vi "ZE_Recorder_InitializeTask.vi"(8 "error in (no error)":errorcluster, 9 "Sampling Rate [Hz]":dbl, 10 "Multi devices?":bool=TRUE, 11 "Channel Array in":T1 caption="Channel Array" {"Terminal" items=["Default"=-1, "RSE"=10083, "NRSE"=10078, "Differential"=10106, "Pseudodifferential"=12529]}) -> (0 "error out":errorcluster, 2 "Array":refnum<k21>[](array[refnum]), 3 "max Range":dbl)   [LabVIEW 2025, in "ZE_Recorder.lvlib"]
doc: "ZE_Recorder_InitializeTask.vi\n----------------------------------------------\nThis VI initalizes the necessary numbers of tasks accrding the number of devices used and assigns a common colck. It returns an array of tasks.\n\nInputs:\n---------------------\n- error in (no error) : Cluster; \n- Sampling Rate [Hz] : DBL; \n- Multi devices? : Boolean; \n- Channel Array : 1DArrayOfCluster; \n\nOutputs:\n---------------------\n- error out : Cluster; \n- Array : 1DArrayOfRefnum; \n- max Range : DBL; \n\n----------------------------------------------\n25.12.2016\nZühlke Engineering AG\nCH-8952 Schlieren\nwww.zuehlke.com"
uses:
  ZE_Recorder.lvlib
  ZE_Recorder_ChannelCluster.ctl
  ChannelCluster.ctl
  ZE_Recorder_Units.ctl
  Temperature.ctl
  <vilib>/DAQmx/configure/timing.llb/DAQmx Timing (Sample Clock).vi
panel:
  # "Connector Pane"
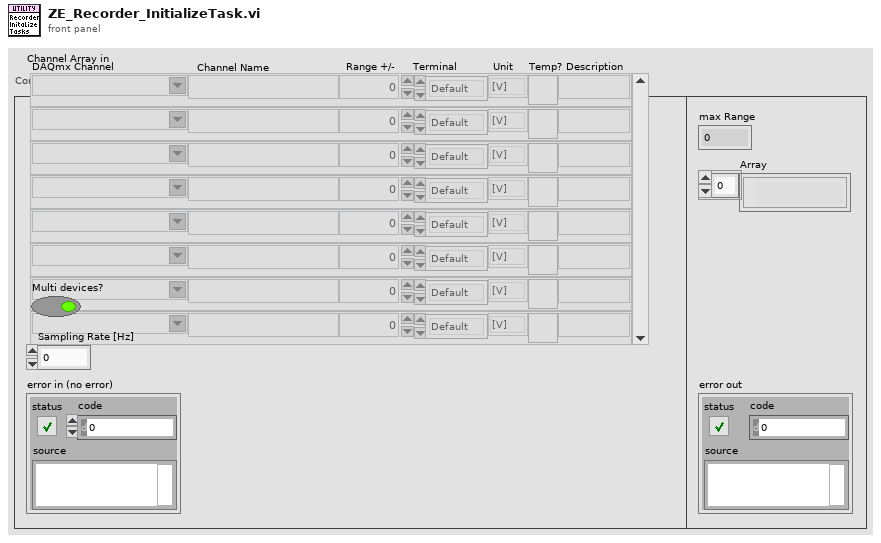
[diagram p1: front panel]
types:
  T1 = typedef "ZE_Recorder.lvlib/ZE_Recorder_ChannelCluster.ctl" = T2[]
  T2 = typedef "ZE_Recorder.lvlib/ChannelCluster.ctl" = cluster{"physical channel":tag, "channel name":string, "Range":dbl, "Terminal":i32, "Unit":T3, "isTemp":T4, "Description":string}
  T3 = typedef "ZE_Recorder.lvlib/ZE_Recorder_Units.ctl" = enum16{"[V]", "[A]", "[F]", "[H]", "[°C]", "[ml/s]", "[m/s]", "[bar]", "[%]", "[N]", "[?]"}
  T4 = typedef "ZE_Recorder.lvlib/Temperature.ctl" = bool
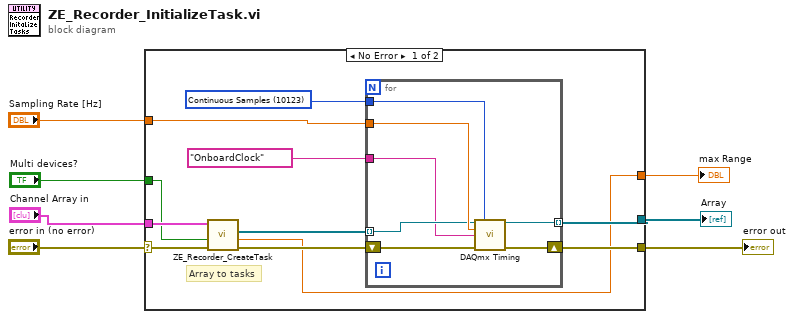
[diagram p0: block diagram]
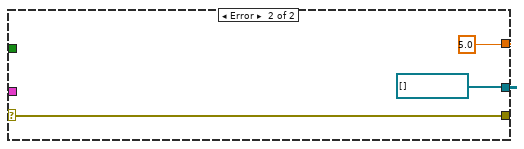
[diagram p2: hidden frame]
diagram:
  n1 = case shown="No Error" "error in (no error)" {
    selector: "error in (no error)" -> [w15 w28]
    tunnel: [w18 refnum<k21>[] []] -> w7
    tunnel: [w13 5.0 ("max Range")] -> w6
    tunnel: "Channel Array in" -> [w11 _]
    tunnel: "Sampling Rate [Hz]" -> [w17 _]
    tunnel: [w16 w28] -> w3
    tunnel: "Multi devices?" -> [w10 _]
    frame No Error {
      w9 = 10123 items=["Finite Samples"=10178, "Continuous Samples"=10123, "Hardware Timed Single Point"=12522] ("sample mode")
      # "Array to tasks"
      n2 = call "ZE_Recorder_CreateTask.vi"("error in"=w15, "multi device"=w10, "Channel Array In"=w11) -> ("error out"=w14:errorcluster, "max Range"=w13:dbl, "Task Array"=w12:refnum<k21>[])  [unwired: 5 in, 1 out]
      n3 = for {
        tunnel: w12 -> [w21] mode=indexing
        shift-right: [w24] -> w16
        shift-left: w14 -> [w25]
        tunnel: [w23] -> w18 mode=indexing
        tunnel: w17 -> [w22]
        tunnel: w9 -> [w20]
        tunnel: tag "OnboardClock" ("source") -> [w19]
        n4 = call-poly <vilib>:"DAQmx Timing.vi"("task/channels in"=w21, "sample mode"=w20, "rate"=w22, "source"=w19, "error in"=w25) -> ("task out"=w23:refnum<k21>, "error out"=w24:errorcluster)  [unwired: 9 in]
      }
    }
    frame Error {
    }
  }
  "Array" <- w7
  "max Range" <- w6
  "error out" <- w3
